vi "习题4.7.vi"   [LabVIEW 2017]
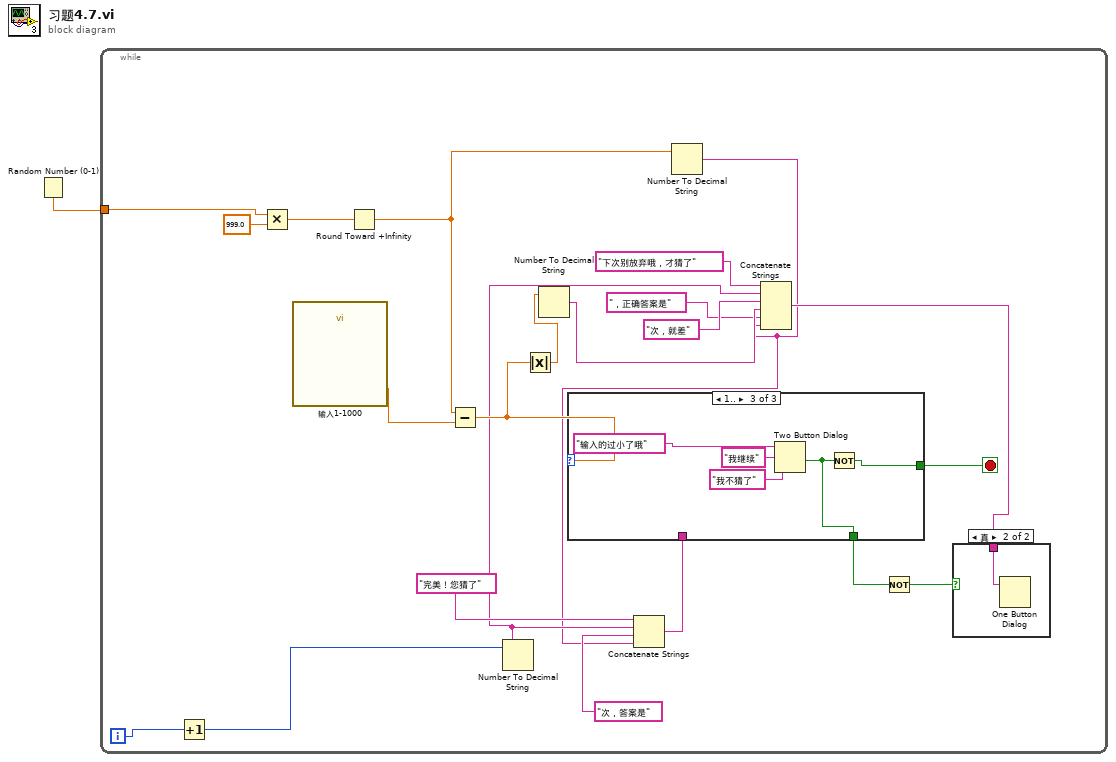
[diagram p0: block diagram]
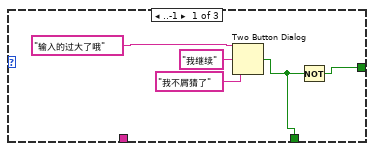
[diagram p3: hidden frame]
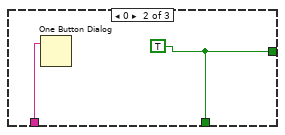
[diagram p4: hidden frame]
diagram:
  n1 = Random Number (0-1)() -> (number: 0 to 1=w1:dbl)
  n2 = while {
    tunnel: w1 -> [w21]
    i -> [w20]
    stop <- w14 stop-if-true
    n3 = Increment(x=w20) -> (x+1=w19:i32)
    n4 = Multiply(x=w21, y=999.0) -> (x*y=w22:dbl)
    n5 = call "输入1-1000"() -> ("1-1000"=w15:dbl)  [unwired: 17 in, 2 out]
    n6 = Round Toward +Infinity(x=w22) -> (ceil(x): smallest int >= x=w3:dbl)
    n7 = Subtract(x=w3, y=w15) -> (x-y=w11:dbl)
    n8 = Number To Decimal String(number=w19) -> (decimal integer string=w7:string)  [unwired: 1 in]
    n9 = Absolute Value(x=w11) -> (abs(x)=w10:dbl)
    n10 = Number To Decimal String(number=w10) -> (decimal integer string=w5:string)  [unwired: 1 in]
    n11 = Number To Decimal String(number=w3) -> (decimal integer string=w2:string)  [unwired: 1 in]
    n12 = Concatenate Strings("完美！您猜了", w7, "次，答案是", w2) -> (w16:string)
    n13 = case shown="1.." w11 {
      tunnel: w16 -> [_ w31 _]
      tunnel: [w26 w30 w33] -> w14
      tunnel: [w25 w30 w32] -> w13
      frame ..-1 {
        n14 = Two Button Dialog(message="输入的过大了哦" ("消息"), 1:"我不屑猜了" ("F按钮名称（“取消”）"), 2:"我继续" ("T按钮名称（“确定”）")) -> (T button?=w25:bool)
        n15 = Not(x=w25) -> (.not. x?=w26:bool)
      }
      frame 0 {
        w30 = TRUE
        n16 = One Button Dialog(message=w31) -> ()  [unwired: 1 in, 1 out]
      }
      frame 1.. {
        n17 = Two Button Dialog(message="输入的过小了哦" ("消息"), 1:"我不猜了" ("F按钮名称（“取消”）"), 2:"我继续" ("T按钮名称（“确定”）")) -> (T button?=w32:bool)
        n18 = Not(x=w32) -> (.not. x?=w33:bool)
      }
    }
    n19 = Concatenate Strings("下次别放弃哦，才猜了" ("消息"), w7, "次，就差" ("字符串"), w5, "，正确答案是" ("字符串"), w2) -> (w8:string)
    n20 = Not(x=w13) -> (.not. x?=w12:bool)
    n21 = case shown="真" w12 {
      tunnel: w8 -> [_ w24]
      frame False {
      }
      frame True {
        n22 = One Button Dialog(message=w24) -> ()  [unwired: 1 in, 1 out]
      }
    }
  }
